vi "DEMO.vi"() -> ()   [LabVIEW 2012, in "Listbox Tool.lvlib"]
uses:
  Listbox Tool.lvlib
panel:
  in  "列表框":i32(listbox)=1
  in  "Items":string[](array[string])
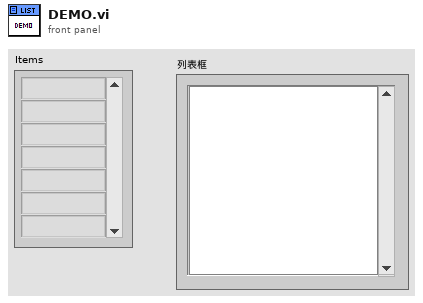
[diagram p1: front panel]
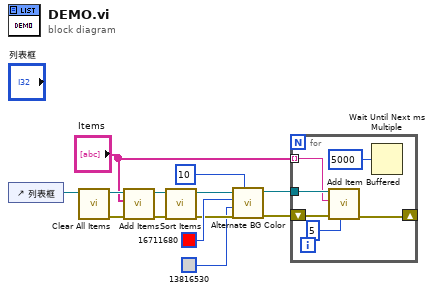
[diagram p0: block diagram]
diagram:
  n1 = control-ref of="列表框"() -> (w9:refnum<vi>)
  n2 = call "Clear All Items.vi"("Listbox Ref"=w9) -> ("错误输出"=w12:errorcluster, "Dup Listbox Ref"=w13:refnum<vi>)  [unwired: 9 in]
  n3 = call "Add Items.vi"("错误输入"=w12, "Items"="Items", "Listbox Ref"=w13) -> ("错误输出"=w10:errorcluster, "Dup Listbox Ref"=w11:refnum<vi>)  [unwired: 7 in]
  n4 = call "Sort Items.vi"("错误输入"=w10, "Listbox Ref"=w11) -> ("错误输出"=w5:errorcluster, "Dup Listbox Ref"=w7:refnum<vi>)  [unwired: 8 in]
  n5 = call "Alternate BG Color.vi"("Number of Rows"=10, "错误输入"=w5, "Second BG Color"=u32 13816530, "First BG Color"=u32 16711680, "Listbox Ref"=w7) -> ("错误输出"=w2:errorcluster, "Dup Listbox Ref"=w3:refnum<vi>)  [unwired: 5 in]
  n6 = for {
    tunnel: w3 -> [w19]
    tunnel: "Items" -> [w16] mode=indexing
    shift-right: [w15] -> _
    shift-left: w2 -> [w18]
    n7 = call "Add Item Buffered.vi"("Items Array Length"=5, "错误输入"=w18, "Item"=w16, "Listbox Ref"=w19) -> ("错误输出"=w15:errorcluster)  [unwired: 6 in, 1 out]
    n8 = Wait Until Next ms Multiple(millisecond multiple=u32 5000 ("毫秒倍数")) -> ()  [unwired: 1 out]
  }
